vi "CapacitiveLevelSensor.vi"() -> ()   [LabVIEW 2022 SP3]
uses:
  <vilib>/DAQmx/read.llb/DAQmx Read (Analog DBL 1Chan 1Samp).vi
  <vilib>/DAQmx/create/channels.llb/DAQmx Create Channel (AI-Voltage-Basic).vi
  <vilib>/DAQmx/miscellaneous.llb/DAQmx Fill In Error Info.vi
  <vilib>/ptbypt/NI_PtbyPt.lvlib
panel:
  out "rms":sgl
  out "Waveform Chart 2":dbl(graph)
  in  "stop":bool
  out "Numeric":dbl
  out "Waveform Chart":dbl(graph)
  in  "DAQmx Physical Channel":tag
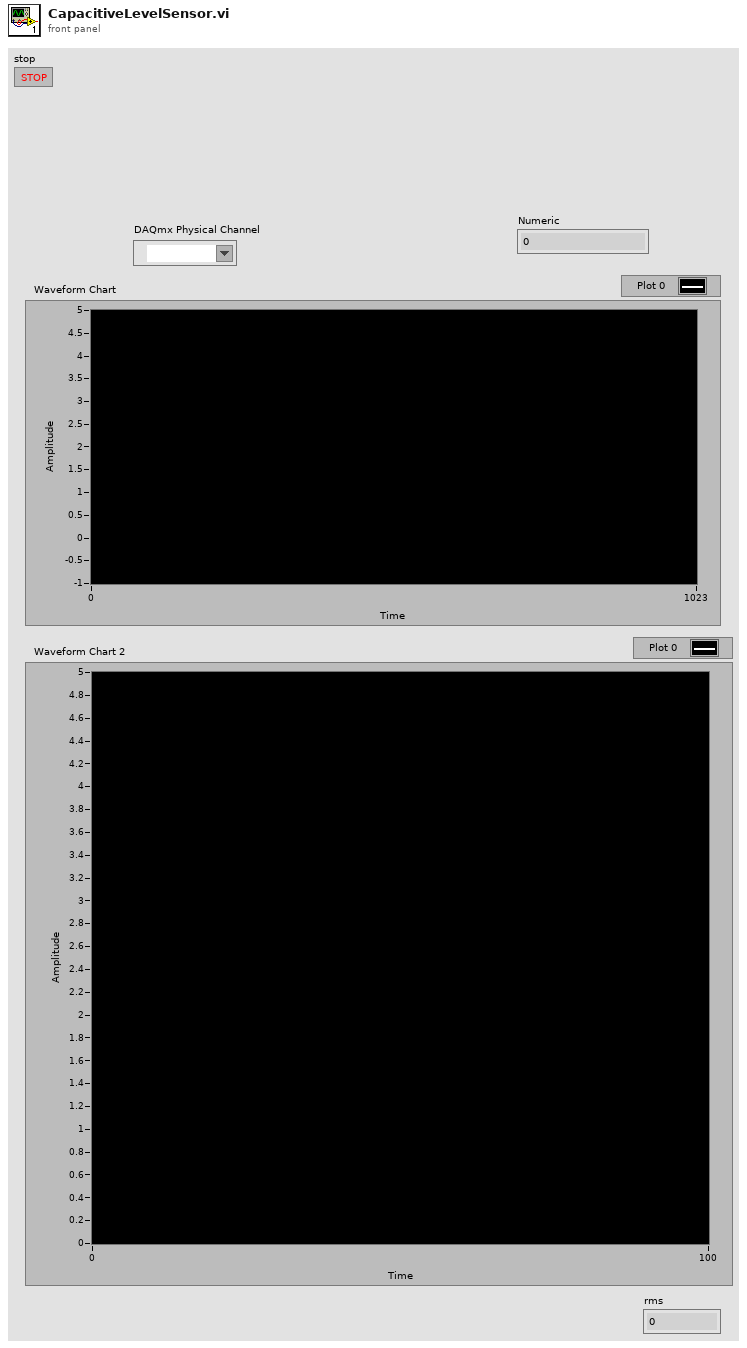
[diagram p1: front panel]
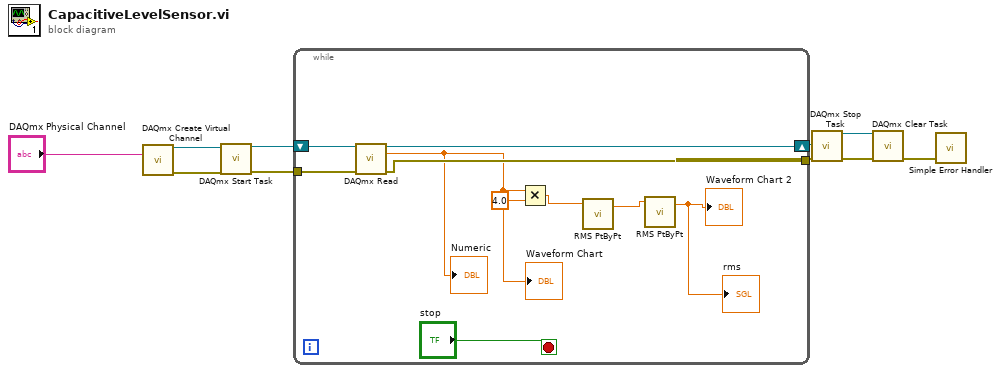
[diagram p0: block diagram]
diagram:
  n1 = call-poly <vilib>:"DAQmx Create Virtual Channel.vi"("physical channels"="DAQmx Physical Channel") -> ("task out"=w10:refnum<k21>, "error out"=w8:errorcluster)  [unwired: 13 in]
  n2 = call <vilib>:"DAQmx Start Task.vi"("task/channels in"=w10, "error in"=w8) -> ("task out"=w9:refnum<k21>, "error out"=w7:errorcluster)  [unwired: 12 in]
  n3 = while {
    tunnel: w7 -> [w19]
    shift-right: [w18] -> w5
    shift-left: w9 -> [w20]
    tunnel: [w16] -> w3
    stop <- "stop" stop-if-true
    n4 = call-poly <vilib>:"DAQmx Read.vi"("task/channels in"=w20, "error in"=w19) -> ("task out"=w18:refnum<k21>, "data"=w14:dbl, "error out"=w16:errorcluster)  [unwired: 11 in]
    "Numeric" <- w14
    "Waveform Chart" <- w14
    n5 = Multiply(x=w14, y=4.0) -> (x*y=w15:dbl)
    n6 = call <vilib>:"RMS PtByPt.vi"("x"=w15) -> ("rms value"=w12:dbl)  [unwired: 3 in, 1 out]
    n7 = call <vilib>:"RMS PtByPt.vi"("x"=w12) -> ("rms value"=→"Waveform Chart 2" →"rms":dbl)  [unwired: 3 in, 1 out]
  }
  n8 = call <vilib>:"DAQmx Stop Task.vi"("task/channels in"=w5, "error in"=w3) -> ("task out"=w2:refnum<k21>, "error out"=w4:errorcluster)  [unwired: 12 in]
  n9 = call <vilib>:"DAQmx Clear Task.vi"("task in"=w2, "error in"=w4) -> ("error out"=w1:errorcluster)  [unwired: 13 in]
  n10 = call <vilib>:"Simple Error Handler.vi"("error in (no error)"=w1) -> ()  [unwired: 4 in, 5 out]
